vi "Initialize.vi"(8 "error in":errorcluster, 11 "Plugin in":refnum<class "StreamWriter.lvclass">) -> (0 "error out":errorcluster, 3 "Plugin out":refnum<class "StreamWriter.lvclass">)   [LabVIEW 2024, in "StreamWriter.lvlib" / "StreamWriter.lvclass"]
uses:
  StreamWriter.lvclass
  C:/Program Files/National Instruments/LabVIEW 2024/vi.lib/FlexLogger/SDK/PluginSDK.lvlibp/PEFClasses/SDK/Plugin/Plugin.lvclass
  <vilib>/FlexLogger/SDK/PluginSDK.lvlibp/PEFClasses/SDK/Processing Element/Timing Parameters.ctl
  <vilib>/FlexLogger/SDK/PluginSDK.lvlibp/PEFClasses/SDK/Processing Element/Timing Method.ctl
  StreamWriter Strings.vi
  <vilib>/FlexLogger/SDK/PluginSDK.lvlibp/PEFClasses/SDK/Plugin/ParameterAccess/Write I32.vi
  <vilib>/FlexLogger/SDK/PluginSDK.lvlibp/PEFClasses/SDK/Plugin/ParameterAccess/Write N Channel.vi
  <vilib>/FlexLogger/SDK/PluginSDK.lvlibp/PEFClasses/SDK/Plugin/Plugin.lvclass
  <vilib>/FlexLogger/SDK/PluginSDK.lvlibp/PEFClasses/SDK/Processing Element/Processing Element.lvclass
  C:/Program Files/National Instruments/LabVIEW 2024/vi.lib/FlexLogger/SDK/PluginSDK.lvlibp/PEFClasses/SDK/Processing Element/Processing Element.lvclass
  C:/Users/Administrator/Documents/LabVIEW Projects/FlexLogger IO Plug-ins/StreamWriter/StreamWriter.lvclass
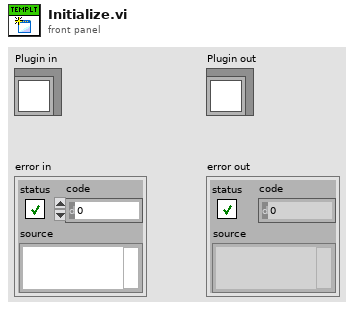
[diagram p1: front panel]
types:
  T1 = typedef "PluginSDK.lvlibp/Processing Element.lvclass/Timing Parameters.ctl" = cluster{"Timing Method":T2, "Timing Period (ms)":i32}
  T2 = typedef "PluginSDK.lvlibp/Processing Element.lvclass/Timing Method.ctl" = enum16{"Periodic", "Immediate", "On Data Ready", "Triggered"}
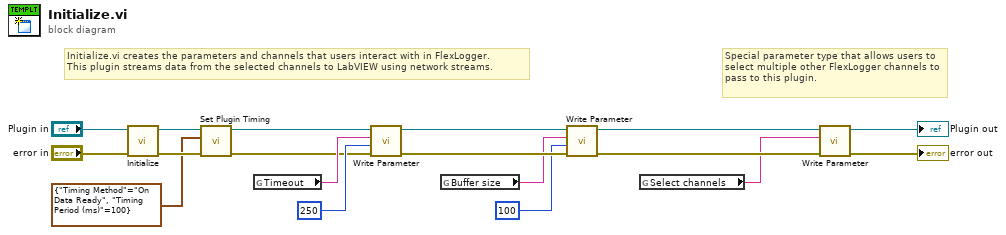
[diagram p0: block diagram]
diagram:
  # "Special parameter type that allows users to select multiple other FlexLogger channels to pass to this plugin."
  # "Initialize.vi creates the parameters and channels that users interact with in FlexLogger.\nThis plugin streams data from the selected channels to LabVIEW using network streams."
  n1 = call-parent "Initialize.vi"("error in (no error)"="error in", "Plugin in"="Plugin in") -> ("error out"=w17:errorcluster, "Plugin out"=w18:refnum<class "StreamWriter.lvclass">)  [unwired: 8 in]
  n2 = call <vilib>:"Set Plugin Timing.vi"("error in (no error)"=w17, "Timing Parameters"=T1 {"Timing Method"=enum."On Data Ready", "Timing Period (ms)"=100}, "Plugin in"=w18) -> ("error out"=w1:errorcluster, "Plugin out"=w2:refnum<class "StreamWriter.lvclass">)  [unwired: 7 in]
  n3 = global read "StreamWriter Strings.vi" "Timeout"() -> (w5:string)
  n4 = call-poly <vilib>:"Write Parameter.vi"("error in (no error)"=w1, "Value"=250, "Name"=w5, "Plugin in"=w2) -> ("error out"=w13:errorcluster, "Plugin out"=w15:refnum<class "StreamWriter.lvclass">)  [unwired: 6 in]
  n5 = global read "StreamWriter Strings.vi" "Buffer size"() -> (w4:string)
  n6 = call-poly <vilib>:"Write Parameter.vi"("error in (no error)"=w13, "Value"=100, "Name"=w4, "Plugin in"=w15) -> ("error out"=w12:errorcluster, "Plugin out"=w14:refnum<class "StreamWriter.lvclass">)  [unwired: 6 in]
  n7 = global read "StreamWriter Strings.vi" "Select channels"() -> (w3:string)
  n8 = call-poly <vilib>:"Write Parameter.vi"("error in (no error)"=w12, "Name (Unique Channel Identifier)"=w3, "Plugin in"=w14) -> ("error out"=→"error out":errorcluster, "Plugin out"=→"Plugin out":refnum<class "StreamWriter.lvclass">)  [unwired: 7 in]
